vi "DAQmx Read (Counter 1D DBL NChan 1Samp).vi"(0 "task/channels in":refnum<k21>, 9 "timeout":dbl=10.0 format="%0.2f", 11 "error in":errorcluster) -> (4 "task out":refnum<k21>, 6 "data":dbl[](array[numeric]) format="%0.2f", 15 "error out":errorcluster)   [LabVIEW 2020]
doc: "Reads one floating-point sample from one or more counter tasks. Use an instance that reads a floating-point value when NI-DAQmx scales counter samples to a floating-point value."
uses:
  nilvaiu.dll
panel:
  # "channel"
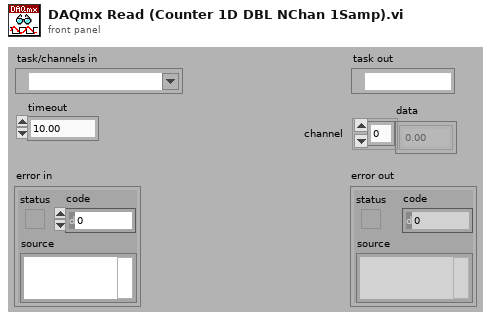
[diagram p1: front panel]
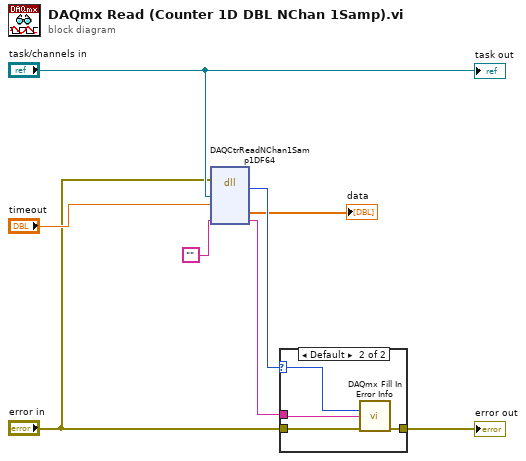
[diagram p0: block diagram]
diagram:
  n1 = dll-call lib="nilvaiu.*" fn="DAQCtrReadNChan1Samp1DF64" ("nilvaiu.*:DAQReadNChan1Samp1DF64_130")(error in="error in", "taskID"="task/channels in", "timeout"="timeout", "extendedErrorInfo"="") -> ("return type"=w6:i32, "data"=→"data":dbl[], "extendedErrorInfo"=w4:string)  [unwired: 4 in, 3 out]
  n2 = case shown="Default" w6 {
    selector: w6 -> [_ w11]
    tunnel: "error in" -> [w9 w13]
    tunnel: [w9 w12] -> w8
    tunnel: w4 -> [_ w10]
    frame 0 {
    }
    frame Default {
      n3 = call "DAQmx Fill In Error Info.vi"("status code"=w11, "extended error info"=w10, "error in"=w13) -> ("error out"=w12:errorcluster)  [unwired: 1 in, 11 out]
    }
  }
  "error out" <- w8
  "task out" <- "task/channels in"
